vi "uService GUI.vi"(8 "error in (no error)":errorcluster, 11 "uService Template in":refnum<class "Father of all uServices.lvclass">) -> (3 "uService Template out":refnum<class "Father of all uServices.lvclass">)   [LabVIEW 2026, in "TALOS.lvlib" / "Father of all uServices.lvlib" / "Father of all uServices.lvclass"]
uses:
  Father of all uServices.lvclass
  C:/LabVIEW Code/TALOS/talos/Ancestor/Ancestor/Ancestor.lvclass
  C:/LabVIEW Code/TALOS/builds/Actor Framework PPL/Actor Framework.lvlibp/1abvi3w/vi.lib/ActorFramework/Actor/Actor.lvclass
  Ancestor/Ancestor/Ancestor.lvclass/Ancestor.ctl
  Classes/uService List/uService List.lvclass/uService List.ctl
  Father of all uServices.lvclass/Father of all uServices.ctl
  builds/Actor Framework PPL/Actor Framework.lvlibp/1abvi3w/vi.lib/ActorFramework/Message Enqueuer/Message Priority.ctl
  Ancestor/Ancestor Messages/Process EH Error Msg/Process EH Error Msg.lvclass/Process EH Error Msg.ctl
  Classes/uService List/Set VI Ref.vi
  Classes/uService List/Set FP Items Refs Maps.vi
  Ancestor/Ancestor/Write uS List Ref.vi
  Support VIs/Generate Error.vi
  FGV/Error Memory/Get Error Description.vi
  Support VIs/Get PC name.vi
  Support VIs/Get Class Name.vi
  FGV/Error Memory/Error Memory Core.vi
  <vilib>/AdvancedString/Delimited String to 1D String Array.vi
  <vilib>/AdvancedString/Delimited String to 1D String Array (string).vi
  Support VIs/Circus Root Path.vi
  FGV/Error Memory/Error Crt Lvl checker.vi
  FGV/Error Memory/Error Memory Core.vi/40c8088d-b597-4017-91af-faa98e00292e.vi
  FGV/Error Memory/Error Memory Core.vi/d4a3ab98-063c-4e44-b43d-fbdcfe6c2be2.vi
  Support VIs/Global Memory.vi
  <vilib>/Utility/LVClass/Get LV Class Name.vi
  Support VIs/Is in Packed Library.vi
  Support VIs/TALOS Root path.vi
  Support VIs/Read CSV worksheet.vi
  Support VIs/Global Constants.vi
  <vilib>/Utility/error.llb/General Error Handler.vi
  <vilib>/Utility/traverseref.llb/TRef Get All FP References.vi
  Support VIs/Error Log.vi
  builds/Actor Framework PPL/Actor Framework.lvlibp/1abvi3w/vi.lib/ActorFramework/Message Enqueuer/Enqueue.vi
  Classes/uService List/uService List.lvclass
  Ancestor/Ancestor/Ancestor.lvclass
  <vilib>/Comparison/Equal/Equal Functor/Equal Functor.lvclass
  Ancestor/Ancestor Messages/Process EH Error Msg/Process EH Error Msg.lvclass
  builds/Actor Framework PPL/Actor Framework.lvlibp/1abvi3w/vi.lib/ActorFramework/Message Enqueuer/Message Enqueuer.lvclass
  builds/Actor Framework PPL/Actor Framework.lvlibp/1abvi3w/vi.lib/ActorFramework/Actor/Actor.lvclass
  TALOS.lvlib
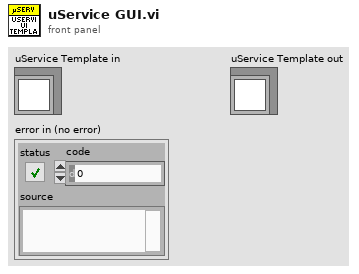
[diagram p1: front panel]
types:
  T1 = typedef "Actor Framework.lvlibp/Message Enqueuer.lvclass/Message Priority.ctl" = enum16{"Low", "Normal", "High"}
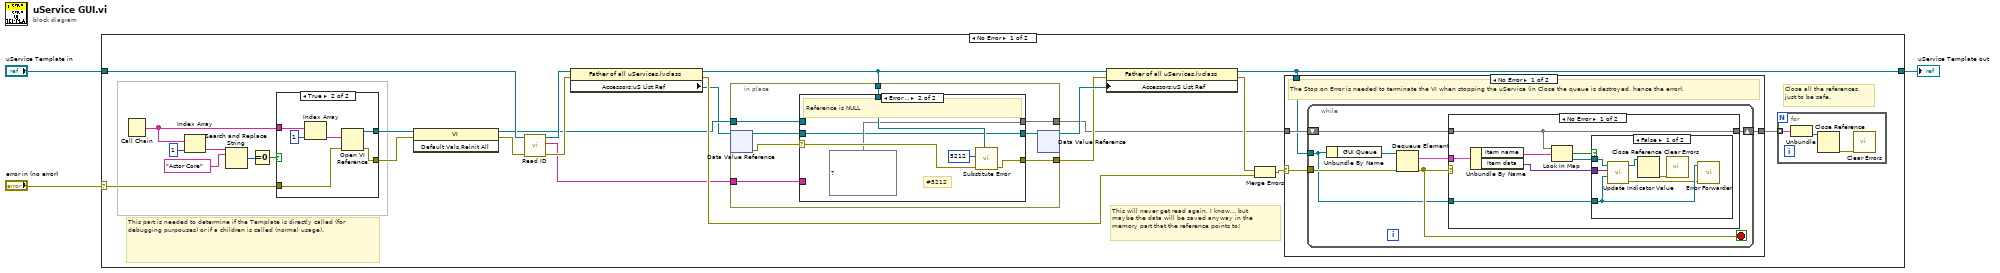
[diagram p0: block diagram]
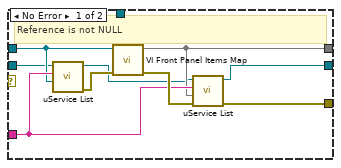
[diagram p2: hidden frame]
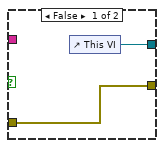
[diagram p3: hidden frame]
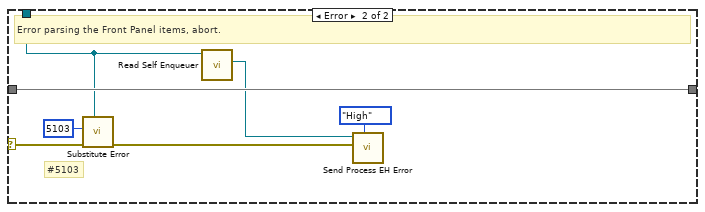
[diagram p6: hidden frame]
diagram:
  n1 = case shown="No Error" "error in (no error)" {
    selector: "error in (no error)" -> [w21 _]
    tunnel: "uService Template in" -> [w14 w95]
    tunnel: [w15 w95] -> w2
    frame No Error {
      # "This will never get read again, I know... but maybe the data will be saved anyway in the memory part that the reference points to!"
      # "This part is needed to determine if the Template is directly called (for debugging purpouses) or if a children is called (normal usage)."
      # "Close all the references, just to be safe."
      n2 = Call Chain() -> (call chain=w22:string[])
      n3 = Index Array(array=w22, index=1) -> (element=w26:string)
      n4 = Search and Replace String(input string=w26, search string="Actor Core" ("regular expression")) -> (number of replacements=w24:i32)  [unwired: 6 in, 3 out]
      n5 = Equal To 0?(x=w24) -> (x = 0?=w23:bool)
      n6 = case shown="True" w23 {
        tunnel: [w53 w56] -> w20
        tunnel: w22 -> [_ w59]
        tunnel: [w52 w55] -> w19
        tunnel: w21 -> [w52 w54]
        frame False {
          n7 = control-ref of="This VI"() -> (w53:refnum<vi>)
        }
        frame True {
          n8 = Index Array(array=w59, index=1) -> (element=w57:string)
          n9 = Open VI Reference(vi path=w57, error in (no error)=w54) -> (vi reference=w56:refnum<vi>, error out=w55:errorcluster)  [unwired: 4 in]
        }
      }
      n10 = invoke class="VI" method="Default Vals.Reinit All"(reference=w20, error in=w19) -> (reference out=w10:refnum<vi>, error out=w18:errorcluster)  [unwired: 1 in, 1 out]
      n11 = call "Read ID.vi"("error in (no error)"=w18, "Ancestor in"=w14) -> ("error out"=w16:errorcluster, "ID"=w8:string, "Ancestor out"=w17:refnum<class "Father of all uServices.lvclass">)  [unwired: 7 in]
      n12 = property class="Father of all uServices.lvclass"(reference=w17, error in=w16) -> (reference out=w4:refnum<class "Father of all uServices.lvclass">, error out=w12:errorcluster, "Accessors:uS List Ref"=w9:refnum<data-value>)
      n13 = in-place {
        in-place-border: [w36] -> w6
        in-place-border: w8 -> [w35]
        in-place-border: [w34] -> w5
        in-place-border: w10 -> [w33]
        in-place-border: w4 -> [w29]
        n14 = in-place-dvr #1(w9) -> (w32:refnum<class "uService List.lvclass">, w30:errorcluster)
        n15 = case shown="Error .." w30 {
          selector: w30 -> [_ w49]
          tunnel: [w44 w48] -> w36
          tunnel: w35 -> [w42 _]
          tunnel: [w41 map{string, refnum<vi>} {} ("Map")] -> w34
          tunnel: w33 -> [w39 _]
          tunnel: w32 -> [w38 w46]
          tunnel: [w37 w46] -> w31
          tunnel: w29 -> [_ w51]
          frame No Error {
            # "Reference is not NULL"
            n16 = call-poly "uService List.vi"("Vi Ref"=w39, "ID"=w42, "uService List in"=w38) -> ("error out"=w45:errorcluster, "uService List out"=w40:refnum<class "uService List.lvclass">)  [unwired: 7 in]
            n17 = call "VI Front Panel Items Map.vi"("error in (no error)"=w45, "VI in"=w39) -> ("error out"=w43:errorcluster, "Map"=w41:map{string, refnum<vi>})  [unwired: 8 in]
            n18 = call-poly "uService List.vi"("error in (no error)"=w43, "FP Items Refs Map"=w41, "ID"=w42, "uService List in"=w40) -> ("error out"=w44:errorcluster, "uService List out"=w37:refnum<class "uService List.lvclass">)  [unwired: 6 in]
          }
          frame Error {
            # "#5212"
            # "Reference is NULL"
            n19 = call "Substitute Error.vi"("LabVIEW Object"=w51, "error in (no error)"=w49, "Error Code"=5212) -> ("error out"=w48:errorcluster)  [unwired: 8 in]
          }
        }
        n20 = in-place-dvr #1(w31) -> (w7:refnum<data-value>)  [unwired: 1 out]
      }
      n21 = property class="Father of all uServices.lvclass"(reference=w4, error in=w6, "Accessors:uS List Ref"=w7) -> (reference out=w15:refnum<class "Father of all uServices.lvclass">, error out=w11:errorcluster)
      n22 = Merge Errors(w11, w12) -> (w13:errorcluster)
      n23 = case shown="No Error" w13 {
        selector: w13 -> [w62 w90]
        tunnel: [w63 w91] -> w28
        tunnel: w5 -> [w61 w91]
        tunnel: w15 -> [w60 w88]
        frame No Error {
          # "The Stop on Error is needed to terminate the VI when stopping the uService (in Close the queue is destroyed, hence the error)."
          n24 = while {
            tunnel: w60 -> [w64]
            shift-right: [w67] -> w63
            shift-left: w61 -> [w68]
            tunnel: w62 -> [w65]
            stop <- w69 stop-if-true
            n25 = Unbundle By Name(w64) -> ("GUI Queue"=w66:refnum<queue>)
            n26 = Dequeue Element(queue=w66, error in (no error)=w65) -> (element=w70:cluster{"Item name":string, "Item data":variant}, error out=w69:errorcluster)  [unwired: 1 in, 2 out]
            n27 = case shown="No Error" w69 {
              tunnel: w70 -> [w77 _]
              tunnel: w68 -> [w73 w84]
              tunnel: [w73 w84] -> w67
              tunnel: w64 -> [w71 _]
              frame No Error {
                n28 = Unbundle By Name(w77) -> ("Item name"=w75:string, "Item data"=w76:variant)
                n29 = Look In Map(map=w73, key=w75) -> (key not found?=w74:bool, value=w72:refnum<vi>)  [unwired: 1 in]
                n30 = case shown="False" w74 {
                  tunnel: w76 -> [w82 _]
                  tunnel: w72 -> [w81 _]
                  tunnel: w71 -> [w80 _]
                  frame False {
                    n31 = call "Update Indicator Value.vi"("uService Template in"=w80, "Item data"=w82, "Control in"=w81) -> ("error out"=w79:errorcluster, "Control out"=w83:refnum<vi>)  [unwired: 7 in]
                    n32 = Close Reference(reference=w83) -> (error out=w78:errorcluster)  [unwired: 1 in]
                    n33 = call <vilib>:"Clear Errors.vi"("error in (no error)"=w78) -> ()  [unwired: 5 in, 2 out]
                    n34 = call "Error Forwarder.vi"("error in (no error)"=w79, "Father of all uServices in"=w80) -> ()  [unwired: 10 in]
                  }
                  frame True {
                  }
                }
              }
              frame Error {
                # "Do nothing"
              }
            }
          }
        }
        frame Error {
          # "#5103"
          # "Error parsing the Front Panel items, abort."
          n35 = call "Substitute Error.vi"("LabVIEW Object"=w88, "error in (no error)"=w90, "Error Code"=5103) -> ("error out"=w86:errorcluster)  [unwired: 8 in]
          n36 = call "Read Self Enqueuer.vi"("Actor"=w88) -> ("Self Enqueuer"=w85:refnum<class "Message Enqueuer.lvclass">)  [unwired: 10 in]
          n37 = call "Send Process EH Error.vi"("Message Priority (Normal)"=Message_Priority."High", "Error to process"=w86, "Message Enqueuer"=w85) -> ()  [unwired: 7 in, 2 out]
        }
      }
      n38 = for {
        tunnel: w28 -> [w94] mode=indexing
        n39 = Unbundle(w94) -> (w93:refnum<vi>)  [unwired: 1 out]
        n40 = Close Reference(reference=w93) -> (error out=w92:errorcluster)  [unwired: 1 in]
        n41 = call <vilib>:"Clear Errors.vi"("error in (no error)"=w92) -> ()  [unwired: 5 in, 2 out]
      }
    }
    frame Error {
    }
  }
  "uService Template out" <- w2
